vi "Test Class EfficientNet_B4.vi"() -> ()   [LabVIEW 2017]
doc: "Created IvanLis by LabVIEW Portal\nProfile: http://labviewportal.org/memberlist.php?mode=viewprofile&u=987\neMail: IvanLisanov@gMail.com\nTelegram: https://t.me/IvanLis"
uses:
  ONNX YOLO Class/ONNX YOLO Class.lvclass
  ONNX Angle Class/ONNX Angle Class.lvclass
  ONNX EfficientNet Class/ONNX EfficientNet Class.lvclass
  ONNX YOLO Class/TypeDef/Circle.ctl
  ONNX YOLO Class/ONNX YOLO Class Library.lvlib
  <vilib>/picture/picture.llb/imagedata.ctl
panel:
  out "Result":T1(array[cluster])
  out "Spin Image":picture[](array[picture])
  out "2D Picture":picture
  out "JPG file path":path=path "/home/ivan/LabVIEWData/ONNX/LabVIEW-ONNX_Runtime/image_for_test/2005mmd_b2_1r_2005mmd_b2_var33.jpg"
  out "error out":errorcluster
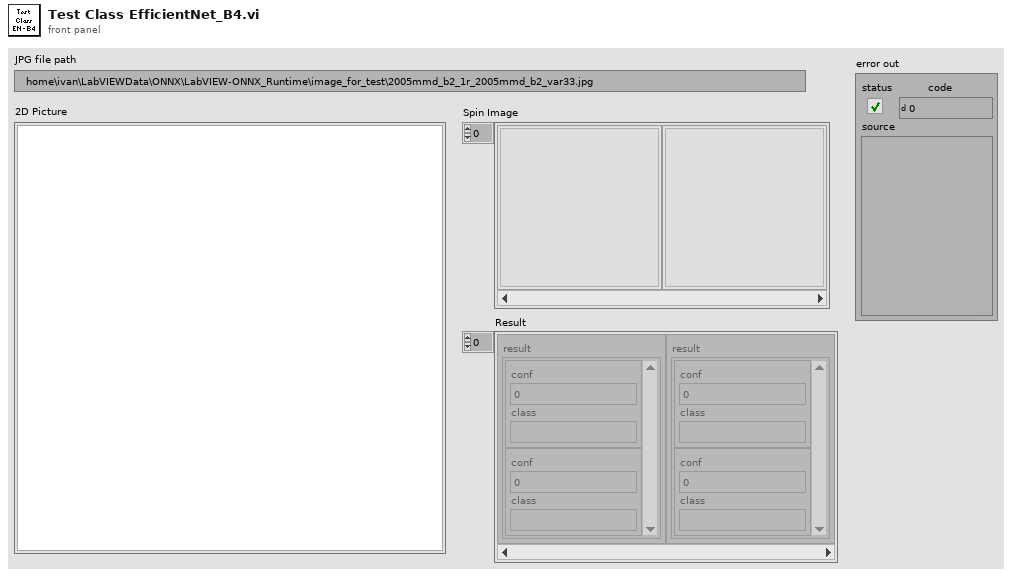
[diagram p1: front panel]
types:
  T1 = cluster{"result":cluster{"conf":sgl, "class":string}[]}[]
  T2 = typedef "ONNX YOLO Class Library.lvlib/Circle.ctl" = cluster{"x":sgl, "y":sgl, "r":sgl}
  T3 = typedef "imagedata.ctl" = cluster{"image type":i32, "image depth":i32, "image":u8[], "mask":u8[], "colors":u32[], "Rectangle":cluster{"left":i16, "top":i16, "right":i16, "bottom":i16}}
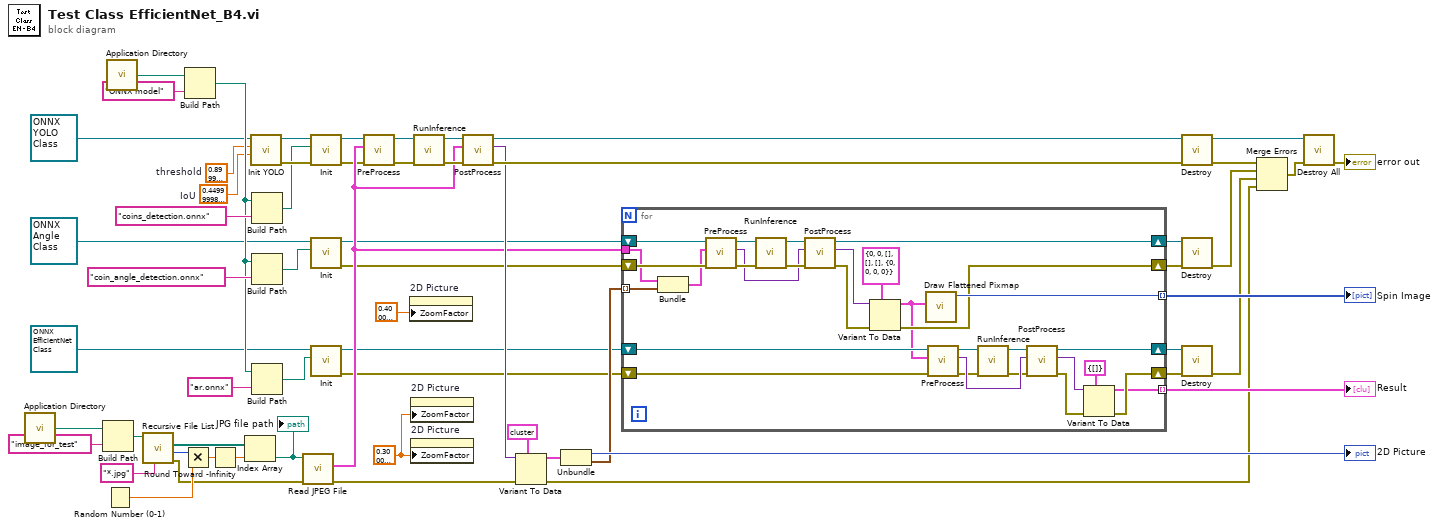
[diagram p0: block diagram]
diagram:
  w44 = sgl 0.45  # IoU
  w45 = sgl 0.9  # threshold
  w60 = sgl 0.3 ("Zoom Factor")
  n1 = call <vilib>:"Application Directory.vi"() -> ("Application Directory"=w51:path)
  n2 = Build Path(base path=w51, name or relative path="image_for_test") -> (appended path=w9:path)
  n3 = Random Number (0-1)() -> (number: 0 to 1=w7:dbl)
  n4 = call <vilib>:"Application Directory.vi"() -> ("Application Directory"=w58:path)
  n5 = call <vilib>:"Recursive File List.vi"("pattern"="*.jpg", "Folder Path"=w9) -> ("error out"=w1:errorcluster, "Number of Files"=w6:i32, "All Files in Dir"=w4:path[])  [unwired: 5 in, 2 out]
  n6 = Multiply(x=w6, y=w7) -> (x*y=w5:dbl)
  n7 = Build Path(base path=w58, name or relative path="ONNX model") -> (appended path=w53:path)
  n8 = Round Toward -Infinity(1:w5) -> (0:w3:dbl)
  n9 = Index Array(array=w4, index=w3) -> (element=w2:path)
  "JPG file path" <- w2
  n10 = call-dynamic "Init YOLO.vi"("IoU"=w44, "threshold"=w45, "ONNX YOLO Class in"=refnum<class "ONNX YOLO Class.lvclass"> refnum) -> ("error out"=w46:errorcluster, "ONNX YOLO Class out"=w47:refnum<class "ONNX YOLO Class.lvclass">)  [unwired: 7 in]
  n11 = Build Path(base path=w53, name or relative path="coins_detection.onnx") -> (appended path=w37:path)
  n12 = Build Path(base path=w53, name or relative path="coin_angle_detection.onnx") -> (appended path=w24:path)
  n13 = Build Path(base path=w53, name or relative path="ar.onnx") -> (appended path=w17:path)
  n14 = call <vilib>:"Read JPEG File.vi"("error in (no error)"=w1, "path to JPEG file"=w2) -> ("error out"=w32:errorcluster, "image data"=w25:T3)  [unwired: 7 in, 1 out]
  n15 = call-dynamic "Init.vi"("error in (no error)"=w46, "ONNX Path"=w37, "ONNX Class in"=w47) -> ("error out"=w22:errorcluster, "ONNX Class out"=w23:refnum<class "ONNX YOLO Class.lvclass">)  [unwired: 6 in, 1 out]
  n16 = call-dynamic "Init.vi"("ONNX Path"=w24, "ONNX Class in"=refnum<class "ONNX Angle Class.lvclass"> refnum ("ONNX Angle Class Library:ONNX Angle Class.lvclass")) -> ("error out"=w20:errorcluster, "ONNX Class out"=w21:refnum<class "ONNX Angle Class.lvclass">)  [unwired: 7 in, 1 out]
  n17 = call-dynamic "Init.vi"("ONNX Path"=w17, "ONNX Class in"=refnum<class "ONNX EfficientNet Class.lvclass"> refnum ("ONNX EfficientNet Class Library:ONNX EfficientNet Class.lvclass")) -> ("error out"=w16:errorcluster, "ONNX Class out"=w18:refnum<class "ONNX EfficientNet Class.lvclass">)  [unwired: 7 in, 1 out]
  n18 = call-dynamic "PreProcess.vi"("error in (no error)"=w22, "Variant in"=w25, "ONNX YOLO Class in"=w23) -> ("error out"=w38:errorcluster, "ONNX YOLO Class out"=w39:refnum<class "ONNX YOLO Class.lvclass">)  [unwired: 6 in, 1 out]
  n19 = property on="2D Picture" class="Pict"("ZoomFactor"=sgl 0.4 ("Zoom Factor")) -> ()  [unwired: 2 in, 2 out]
  n20 = property on="2D Picture" class="Pict"("ZoomFactor"=w60) -> ()  [unwired: 2 in, 2 out]
  n21 = property on="2D Picture" class="Pict"("ZoomFactor"=w60) -> ()  [unwired: 2 in, 2 out]
  n22 = call-dynamic "RunInference.vi"("error in (no error)"=w38, "ONNX Class in"=w39) -> ("error out"=w42:errorcluster, "ONNX Class out"=w43:refnum<class "ONNX YOLO Class.lvclass">)  [unwired: 7 in, 1 out]
  n23 = call-dynamic "PostProcess.vi"("error in (no error)"=w42, "Variant in"=w25, "ONNX YOLO Class in"=w43) -> ("error out"=w40:errorcluster, "Variant out"=w33:variant, "ONNX YOLO Class out"=w41:refnum<class "ONNX YOLO Class.lvclass">)  [unwired: 6 in]
  n24 = Variant To Data(error in=w32, type=cluster{"new picture":picture, T2[]} {"new picture"=bytes[0], []} ("output cluster"), Variant=w33) -> (data=w34:cluster{"new picture":picture, T2[]}, error out=w11:errorcluster)
  n25 = Unbundle(w34) -> ("new picture"=→"2D Picture":picture, w30:T2[])
  n26 = for {
    tunnel: w30 -> [w82] mode=indexing
    tunnel: [w91] -> w59 mode=indexing
    shift-right: [w84] -> w28
    shift-left: w21 -> [w86]
    shift-right: [w76] -> w27
    shift-left: w20 -> [w85]
    tunnel: w25 -> [w83]
    shift-right: [w63] -> w14
    shift-left: w16 -> [w70]
    shift-right: [w68] -> w15
    shift-left: w18 -> [w69]
    tunnel: [w62] -> w12 mode=indexing
    n27 = Bundle("image data"=w83, "Circle"=w82) -> (w81:cluster{"image data":T3, "Circle":T2})  [unwired: 1 in]
    n28 = call-dynamic "PreProcess.vi"("error in (no error)"=w85, "Variant in"=w81, "ONNX Angle Class in"=w86) -> ("error out"=w87:errorcluster, "Variant out"=w79:variant, "ONNX Angle Class out"=w88:refnum<class "ONNX Angle Class.lvclass">)  [unwired: 6 in]
    n29 = call-dynamic "RunInference.vi"("error in (no error)"=w87, "ONNX Class in"=w88) -> ("error out"=w89:errorcluster, "ONNX Class out"=w90:refnum<class "ONNX Angle Class.lvclass">)  [unwired: 7 in, 1 out]
    n30 = call-dynamic "PostProcess.vi"("error in (no error)"=w89, "Variant in"=w79, "ONNX Angle Class in"=w90) -> ("error out"=w77:errorcluster, "Variant out"=w78:variant, "ONNX Angle Class out"=w84:refnum<class "ONNX Angle Class.lvclass">)  [unwired: 6 in]
    n31 = Variant To Data(error in=w77, type=T3 {"image type"=0, "image depth"=0, "image"=[], "mask"=[], "colors"=[], "Rectangle"={"left"=0, "top"=0, "right"=0, "bottom"=0}} ("image data OUT"), Variant=w78) -> (data=w67:T3, error out=w76:errorcluster)
    n32 = call <vilib>:"Draw Flattened Pixmap.vi"("image data"=w67) -> ("new picture"=w91:picture)  [unwired: 8 in]
    n33 = call-dynamic "PreProcess.vi"("error in (no error)"=w70, "Variant in"=w67, "ONNX EfficientNet Class in"=w69) -> ("error out"=w74:errorcluster, "Variant out"=w75:variant, "ONNX EfficientNet Class out"=w73:refnum<class "ONNX EfficientNet Class.lvclass">)  [unwired: 6 in]
    n34 = call-dynamic "RunInference.vi"("error in (no error)"=w74, "ONNX Class in"=w73) -> ("error out"=w72:errorcluster, "ONNX Class out"=w71:refnum<class "ONNX EfficientNet Class.lvclass">)  [unwired: 7 in, 1 out]
    n35 = call-dynamic "PostProcess.vi"("error in (no error)"=w72, "Variant in"=w75, "ONNX EfficientNet Class in"=w71) -> ("error out"=w66:errorcluster, "Variant out"=w65:variant, "ONNX EfficientNet Class out"=w68:refnum<class "ONNX EfficientNet Class.lvclass">)  [unwired: 6 in]
    n36 = Variant To Data(error in=w66, type=cluster{cluster{"conf":sgl, "class":string}[]} {[]} ("output cluster"), Variant=w65) -> (data=w62:cluster{cluster{"conf":sgl, "class":string}[]}, error out=w63:errorcluster)
  }
  "Spin Image" <- w59
  "Result" <- w12
  n37 = call-dynamic "Destroy.vi"("error in (no error)"=w40, "ONNX Class in"=w41) -> ("error out"=w49:errorcluster, "ONNX Class out"=w50:refnum<class "ONNX YOLO Class.lvclass">)  [unwired: 8 in]
  n38 = call-dynamic "Destroy.vi"("error in (no error)"=w27, "ONNX Class in"=w28) -> ("error out"=w26:errorcluster)  [unwired: 8 in, 1 out]
  n39 = call-dynamic "Destroy.vi"("error in (no error)"=w14, "ONNX Class in"=w15) -> ("error out"=w13:errorcluster)  [unwired: 8 in, 1 out]
  n40 = Merge Errors(w49, w26, w13, w11) -> (w36:errorcluster)
  n41 = call-dynamic "Destroy All.vi"("error in (no error)"=w36, "ONNX Class in"=w50) -> ("error out"=→"error out":errorcluster)  [unwired: 8 in, 1 out]
